vi "c DMC60C Create2.vi"(7 "encoderTicks":i32, 8 "error in (no error)":errorcluster, 9 "gearRatio":dbl, 10 "wheelDiametermm":dbl, 11 "deviceNumber":u8) -> (0 "error out":errorcluster, 3 "function return":i32)   [LabVIEW 2018, in "DMC60C.lvlib"]
doc: "Create a DMC60 Object in memory.\n\n<B>deviceNumber</B> - Device number of the DMC60C.\n<B>wheelDiametermm</B> - The diameter of the wheel in millimeters.\n<B>gearRatio</B> - The ratio of the gearbox (12.75:1 would be 12.75). This should be 1 if the encoder is on the output of the gearbox.\n<B>encoderTicks</B> - The cycles per channel per rotation of the encoder."
uses:
  <vilib>/Rock Robotics/WPI/ThirdParty/TopLevel/DMC60C/DMC60C.lvlib
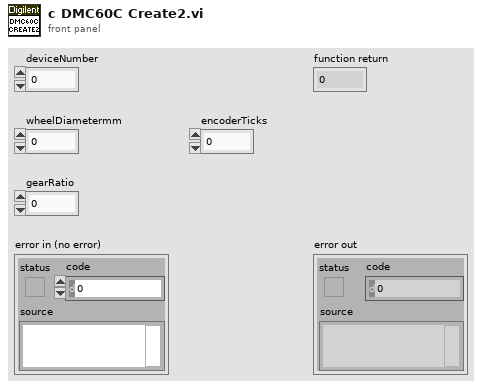
[diagram p1: front panel]
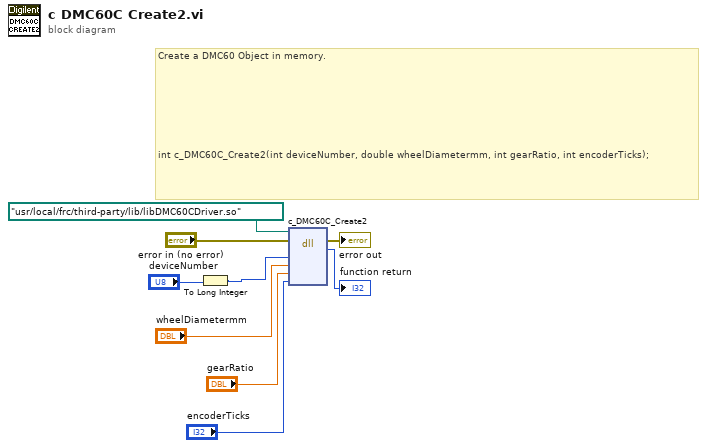
[diagram p0: block diagram]
diagram:
  # "Create a DMC60 Object in memory.\n\n\n\n\n\n\n\n\nint c_DMC60C_Create2(int deviceNumber, double wheelDiametermm, int gearRatio, int encoderTicks);"
  n1 = To Long Integer(number="deviceNumber") -> (32bit integer=w3:i32)
  n2 = dll-call lib="usr/lib/libdmc60c.so" fn="c_DMC60C_Create2"(path in=path "/usr/local/frc/third-party/lib/libDMC60CDriver.so", error in="error in (no error)", "deviceNumber"=w3, "wheelDiametermm"="wheelDiametermm", "gearRatio"="gearRatio", "encoderTicks"="encoderTicks") -> (error out=→"error out":errorcluster, "return type"=→"function return":i32)  [unwired: 5 in, 1 out]
